vi "Configure Log File Properties.vi"(8 "error in (no error)":errorcluster, 9 "Log File Path":string[](array[string]), 10 "File Section Name":string="Log File", 11 "Device Ref in":T1=18446744073709551615 format="%.0x") -> (0 "error out":errorcluster, 3 "Device Ref out":T1 format="%.0x")   [LabVIEW 2019, in "Telemetry System Explorer.lvlib"]
uses:
  Telemetry System Explorer.lvlib
  <vilib>/NI VeriStand/Custom Device API/Custom Device Item Ref.ctl
  <vilib>/NI VeriStand/Custom Device API/Custom Device Channel.ctl
  <vilib>/NI VeriStand/Custom Device API/Custom Device Channel Type.ctl
  Shared/Constants.vi
  <vilib>/NI VeriStand/Custom Device API/Set Item Property (String Array).vi
  <vilib>/NI VeriStand/Custom Device API/Set Item Property (Boolean).vi
  <vilib>/NI VeriStand/Custom Device API/Custom Device API.lvlib
  Shared/Telemetry Shared.lvlib
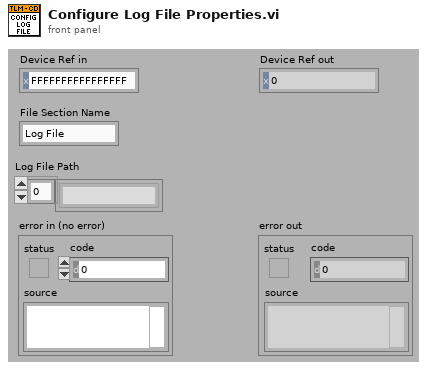
[diagram p1: front panel]
types:
  T1 = typedef "Custom Device API.lvlib/Custom Device Item Ref.ctl" = u64
  T2 = typedef "Custom Device API.lvlib/Custom Device Channel.ctl" = cluster{"Type":T3, "Units":string, "Default Value":dbl, "Faultable":bool, "Scalable":bool}
  T3 = typedef "Custom Device API.lvlib/Custom Device Channel Type.ctl" = enum16{"Input", "Output"}
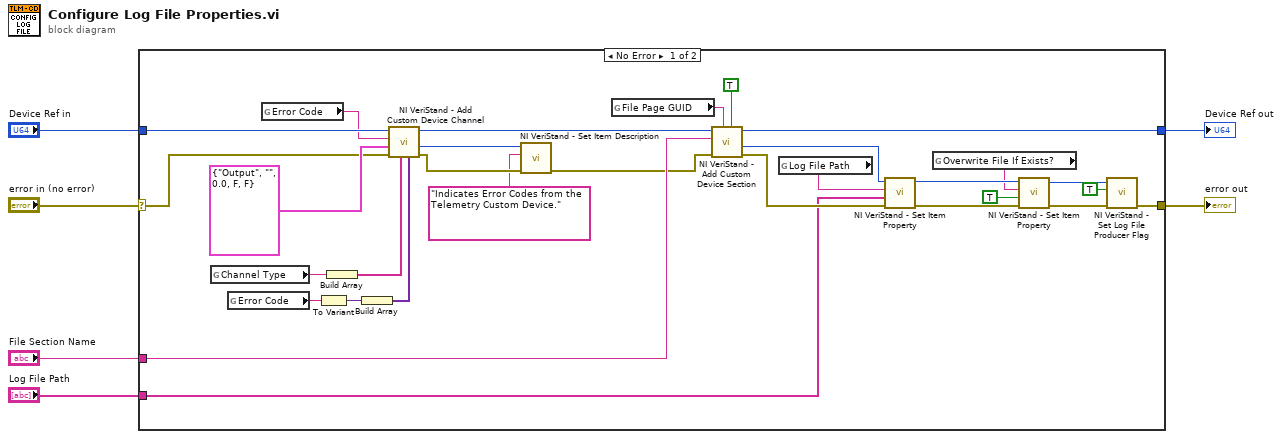
[diagram p0: block diagram]
diagram:
  n1 = case shown="No Error" "error in (no error)" {
    selector: "error in (no error)" -> [w12 w37]
    tunnel: "File Section Name" -> [w35 _]
    tunnel: "Log File Path" -> [w28 _]
    tunnel: "Device Ref in" -> [w14 w38]
    tunnel: [w18 w38] -> w3
    tunnel: [w15 w37] -> w2
    frame No Error {
      n2 = global read "Constants.vi" "Channel Type"() -> (w9:string)
      n3 = global read "Constants.vi" "Error Code"() -> (w7:string)
      n4 = global read "Constants.vi" "Error Code"() -> (w10:string)
      n5 = To Variant(anything=w7) -> (Variant=w20:variant)
      n6 = Build Array(w9) -> (w8:string[])
      n7 = Build Array(w20) -> (w19:variant[])
      n8 = call <vilib>:"NI VeriStand - Add Custom Device Channel.vi"("Property Values"=w19, "Property names"=w8, "error in (no error)"=w12, "Channel"=T2 {"Type"=enum."Output", "Units"="", "Default Value"=0.0, "Faultable"=FALSE, "Scalable"=FALSE}, "Channel Name"=w10, "Parent Ref in"=w14) -> ("error out"=w24:errorcluster, "Channel Ref"=w22:T1, "Parent Ref out"=w13:T1)  [unwired: 2 in, 1 out]
      n9 = call <vilib>:"NI VeriStand - Set Item Description.vi"("error in (no error)"=w24, "Description"="Indicates Error Codes from the Telemetry Custom Device.", "Item Ref in"=w22) -> ("error out"=w11:errorcluster)  [unwired: 6 in, 2 out]
      n10 = global read "Constants.vi" "File Page GUID"() -> (w27:string)
      n11 = call <vilib>:"NI VeriStand - Add Custom Device Section.vi"("Highlight? (F)"=TRUE, "GUID (Default Section)"=w27, "error in (no error)"=w11, "Section Name"=w35, "Parent Ref in"=w13) -> ("error out"=w36:errorcluster, "Section Ptr"=w30:T1, "Parent Ref out"=w18:T1)  [unwired: 2 in, 2 out]
      n12 = global read "Constants.vi" "Log File Path"() -> (w26:string)
      n13 = call-poly <vilib>:"NI VeriStand - Set Item Property.vi"("error in (no error)"=w36, "Value"=w28, "Property Name"=w26, "Item Ref in"=w30) -> ("error out"=w33:errorcluster, "Item Ref out"=w34:T1)  [unwired: 6 out]
      n14 = global read "Constants.vi" "Overwrite File If Exists?"() -> (w25:string)
      n15 = call-poly <vilib>:"NI VeriStand - Set Item Property.vi"("error in (no error)"=w33, "Value"=TRUE, "Property Name"=w25, "Item Ref in"=w34) -> ("error out"=w16:errorcluster, "Item Ref out"=w17:T1)  [unwired: 6 out]
      n16 = call <vilib>:"NI VeriStand - Set Log File Producer Flag.vi"("error in (no error)"=w16, "Log File Producer"=TRUE ("Log File Provider"), "Item Ref in"=w17) -> ("error out"=w15:errorcluster)  [unwired: 7 in, 1 out]
    }
    frame Error {
    }
  }
  "Device Ref out" <- w3
  "error out" <- w2
